vi "SET.vi"(6 "value":string, 8 "error in (no error)":errorcluster, 9 "options":T1={"ms timeout"=-1, "expire time"=timestamp(0 s since 1904-01-01), "NX"=FALSE, "XX"=FALSE, "KEEPTTL"=FALSE, "GET"=FALSE}, 10 "key":string, 11 "Redis Client in":refnum<class "Redis Client.lvclass">) -> (0 "error out":errorcluster, 1 "response":variant, 3 "Redis Client out":refnum<class "Redis Client.lvclass">)   [LabVIEW 2019, in "Redis Client for LabVIEW.lvlib" / "Redis Client.lvclass"]
uses:
  Redis Client.lvclass
  RESP3 for LabVIEW/RESP3/subVIs/RESP3 Make String Base.vi
  RESP3 for LabVIEW/RESP3/types/RESP3 data type attribute.vi
  RESP3 for LabVIEW/RESP3/high-level/RESP3 Get String.vi
  RESP3 for LabVIEW/RESP3/RESP3.lvlib
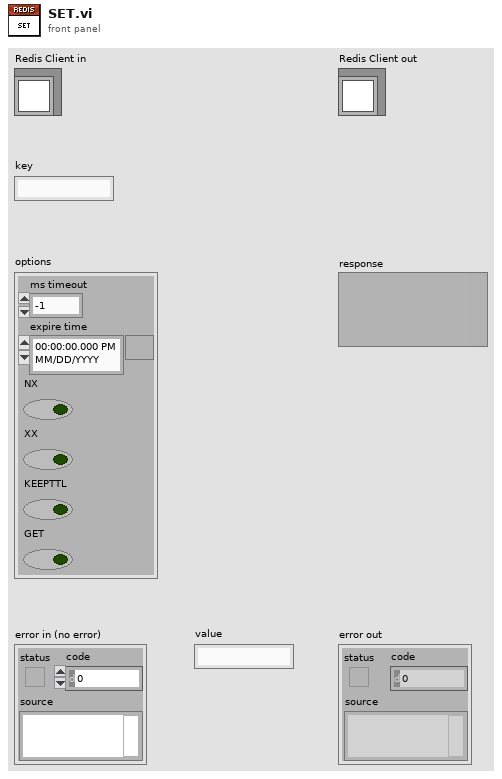
[diagram p1: front panel]
types:
  T1 = cluster{"ms timeout":i64, "expire time":timestamp, "NX":bool, "XX":bool, "KEEPTTL":bool, "GET":bool}
  T2 = typedef "RESP3.lvlib/RESP3 Type.ctl" = enum8{"<0x00>", "<0x01>", "<0x02>", "<0x03>", "<0x04>", "<0x05>", "<0x06>", "<0x07>", "<0x08>", "<0x09>", "<0x0A>", "<0x0B>", "<0x0C>", "<0x0D>", "<0x0E>", "<0x0F>", "<0x10>", "<0x11>", "<0x12>", "<0x13>", "<0x14>", "<0x15>", "<0x16>", "<0x17>", "<0x18>", "<0x19>", "<0x1A>", "<0x1B>", "<0x1C>", "<0x1D>", "<0x1E>", "<0x1F>", "\" \"", "BLOB ERROR", "\"\"\"", "BOOLEAN", "BLOB", "MAP", "\"&\"", "\"'\"", "BIG NUMBER", "\")\"", "ARRAY", "STRING", "DOUBLE", "ERROR", "END", "\"/\"", "\"0\"", "\"1\"", "\"2\"", "\"3\"", "\"4\"", "\"5\"", "\"6\"", "\"7\"", "\"8\"", "\"9\"", "INTEGER", "STREAM", "\"<\"", "VERBATIM STRING", "PUSH", "\"?\"", "\"@\"", "\"A\"", "\"B\"", "\"C\"", "\"D\"", "\"E\"", "\"F\"", "\"G\"", "\"H\"", "\"I\"", "\"J\"", "\"K\"", "\"L\"", "\"M\"", "\"N\"", "\"O\"", "\"P\"", "\"Q\"", "\"R\"", "\"S\"", "\"T\"", "\"U\"", "\"V\"", "\"W\"", "\"X\"", "\"Y\"", "\"Z\"", "\"[\"", "\"\\\"", "\"]\"", "\"^\"", "NULL", "\"`\"", "\"a\"", "\"b\"", "\"c\"", "\"d\"", "\"e\"", "\"f\"", "\"g\"", "\"h\"", "\"i\"", "\"j\"", "\"k\"", "\"l\"", "\"m\"", "\"n\"", "\"o\"", "\"p\"", "\"q\"", "\"r\"", "\"s\"", "\"t\"", "\"u\"", "\"v\"", "\"w\"", "\"x\"", "\"y\"", "\"z\"", "\"{\"", "ATTRIBUTES", "\"}\"", "SET", "<0x7F>", "<0x80>", "<0x81>", "<0x82>", "<0x83>", "<0x84>", "<0x85>", "<0x86>", "<0x87>", "<0x88>", "<0x89>", "<0x8A>", "<0x8B>", "<0x8C>", "<0x8D>", "<0x8E>", "<0x8F>", "<0x90>", "<0x91>", "<0x92>", "<0x93>", "<0x94>", "<0x95>", "<0x96>", "<0x97>", "<0x98>", "<0x99>", "<0x9A>", "<0x9B>", "<0x9C>", "<0x9D>", "<0x9E>", "<0x9F>", "<0xA0>", "<0xA1>", "<0xA2>", "<0xA3>", "<0xA4>", "<0xA5>", "<0xA6>", "<0xA7>", "<0xA8>", "<0xA9>", "<0xAA>", "<0xAB>", "<0xAC>", "<0xAD>", "<0xAE>", "<0xAF>", "<0xB0>", "<0xB1>", "<0xB2>", "<0xB3>", "<0xB4>", "<0xB5>", "<0xB6>", "<0xB7>", "<0xB8>", "<0xB9>", "<0xBA>", "<0xBB>", "<0xBC>", "<0xBD>", "<0xBE>", "<0xBF>", "<0xC0>", "<0xC1>", "<0xC2>", "<0xC3>", "<0xC4>", "<0xC5>", "<0xC6>", "<0xC7>", "<0xC8>", "<0xC9>", "<0xCA>", "<0xCB>", "<0xCC>", "<0xCD>", "<0xCE>", "<0xCF>", "<0xD0>", "<0xD1>", "<0xD2>", "<0xD3>", "<0xD4>", "<0xD5>", "<0xD6>", "<0xD7>", "<0xD8>", "<0xD9>", "<0xDA>", "<0xDB>", "<0xDC>", "<0xDD>", "<0xDE>", "<0xDF>", "<0xE0>", "<0xE1>", "<0xE2>", "<0xE3>", "<0xE4>", "<0xE5>", "<0xE6>", "<0xE7>", "<0xE8>", "<0xE9>", "<0xEA>", "<0xEB>", "<0xEC>", "<0xED>", "<0xEE>", "<0xEF>", "<0xF0>", "<0xF1>", "<0xF2>", "<0xF3>", "<0xF4>", "<0xF5>", "<0xF6>", "<0xF7>", "<0xF8>", "<0xF9>", "<0xFA>", "<0xFB>", "<0xFC>", "<0xFD>", "<0xFE>"}
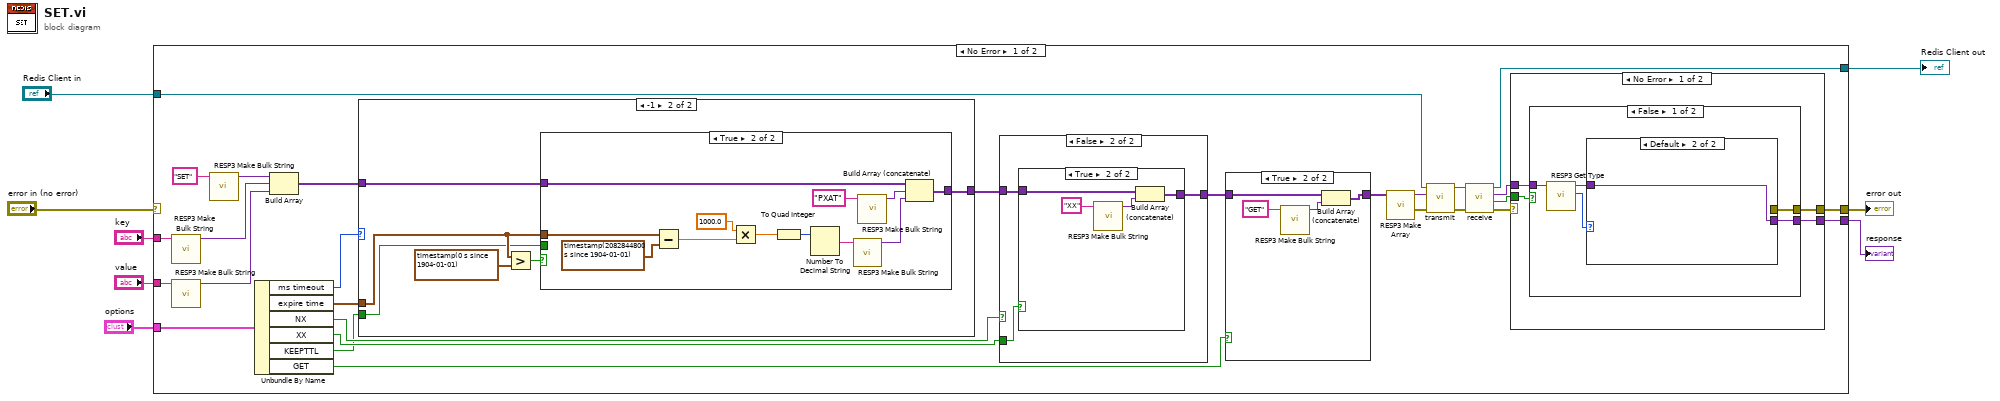
[diagram p0: block diagram]
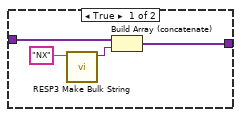
[diagram p3: hidden frame]
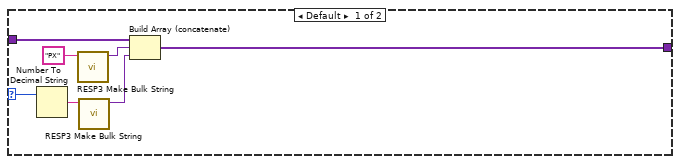
[diagram p5: hidden frame]
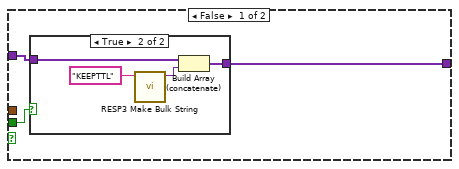
[diagram p6: hidden frame]
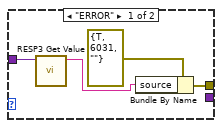
[diagram p8: hidden frame]
diagram:
  n1 = case shown="No Error" "error in (no error)" {
    selector: "error in (no error)" -> [_ w103]
    tunnel: [w29 w103] -> w7
    tunnel: "Redis Client in" -> [w36 w102]
    tunnel: [w34 w102] -> w5
    tunnel: "key" -> [w26 _]
    tunnel: [w28 _] -> w3
    tunnel: "value" -> [w21 _]
    tunnel: "options" -> [w19 _]
    frame No Error {
      n2 = call "RESP3 Make Bulk String.vi"("String"=w26) -> ("RESP3 Value out"=w24:variant)  [unwired: 9 in, 1 out]
      n3 = call "RESP3 Make Bulk String.vi"("String"=w21) -> ("RESP3 Value out"=w20:variant)  [unwired: 9 in, 1 out]
      n4 = call "RESP3 Make Bulk String.vi"("String"="SET" ("string in")) -> ("RESP3 Value out"=w25:variant)  [unwired: 9 in, 1 out]
      n5 = Unbundle By Name(w19) -> ("ms timeout"=w18:i64, "expire time"=w17:timestamp, "NX"=w15:bool, "XX"=w13:bool, "KEEPTTL"=w12:bool, "GET"=w10:bool)
      n6 = Build Array(w25, w24, w20) -> (w16:variant[])
      n7 = case shown="-1" w18 {
        selector: w18 -> [w56 _]
        tunnel: w17 -> [_ w64]
        tunnel: w16 -> [w59 w63]
        tunnel: [w54 w62] -> w14
        tunnel: w12 -> [_ w61]
        frame Default {
          n8 = Number To Decimal String(number=w56) -> (decimal integer string=w55:string)  [unwired: 1 in]
          n9 = call "RESP3 Make Bulk String.vi"("String"="PX") -> ("RESP3 Value out"=w57:variant)  [unwired: 9 in, 1 out]
          n10 = call "RESP3 Make Bulk String.vi"("String"=w55) -> ("RESP3 Value out"=w60:variant)  [unwired: 9 in, 1 out]
          n11 = Build Array (concatenate)(w59, w57, w60) -> (w54:variant[])
        }
        frame -1 {
          n12 = Greater?(x=w64, y=timestamp(0 s since 1904-01-01)) -> (0:w65:bool)
          n13 = case shown="True" w65 {
            tunnel: w64 -> [_ w85]
            tunnel: w63 -> [w68 w79]
            tunnel: [w67 w78] -> w62
            tunnel: w61 -> [w69 _]
            frame False {
              n14 = case shown="True" w69 {
                tunnel: w68 -> [w70 w72]
                tunnel: [w70 w71] -> w67
                frame False {
                }
                frame True {
                  n15 = call "RESP3 Make Bulk String.vi"("String"="KEEPTTL") -> ("RESP3 Value out"=w74:variant)  [unwired: 9 in, 1 out]
                  n16 = Build Array (concatenate)(w72, w74) -> (w71:variant[])
                }
              }
            }
            frame True {
              n17 = Subtract(x=w85, y=timestamp(2082844800 s since 1904-01-01)) -> (x-y=w84:dbl)
              n18 = Multiply(x=1000.0, y=w84) -> (x*y=w82:dbl)
              n19 = To Quad Integer(1:w82) -> (0:w75:i64)
              n20 = Number To Decimal String(number=w75) -> (decimal integer string=w81:string)  [unwired: 1 in]
              n21 = call "RESP3 Make Bulk String.vi"("String"=w81) -> ("RESP3 Value out"=w76:variant)  [unwired: 9 in, 1 out]
              n22 = call "RESP3 Make Bulk String.vi"("String"="PXAT") -> ("RESP3 Value out"=w77:variant)  [unwired: 9 in, 1 out]
              n23 = Build Array (concatenate)(w79, w77, w76) -> (w78:variant[])
            }
          }
        }
      }
      n24 = case shown="False" w15 {
        tunnel: w14 -> [w45 w48]
        tunnel: w13 -> [_ w46]
        tunnel: [w42 w47] -> w11
        frame True {
          n25 = call "RESP3 Make Bulk String.vi"("String"="NX") -> ("RESP3 Value out"=w43:variant)  [unwired: 9 in, 1 out]
          n26 = Build Array (concatenate)(w45, w43) -> (w42:variant[])
        }
        frame False {
          n27 = case shown="True" w46 {
            tunnel: w48 -> [w49 w53]
            tunnel: [w49 w50] -> w47
            frame False {
            }
            frame True {
              n28 = call "RESP3 Make Bulk String.vi"("String"="XX") -> ("RESP3 Value out"=w51:variant)  [unwired: 9 in, 1 out]
              n29 = Build Array (concatenate)(w53, w51) -> (w50:variant[])
            }
          }
        }
      }
      n30 = case shown="True" w10 {
        tunnel: w11 -> [w37 w39]
        tunnel: [w37 w38] -> w9
        frame False {
        }
        frame True {
          n31 = call "RESP3 Make Bulk String.vi"("String"="GET") -> ("RESP3 Value out"=w41:variant)  [unwired: 9 in, 1 out]
          n32 = Build Array (concatenate)(w39, w41) -> (w38:variant[])
        }
      }
      n33 = call "RESP3 Make Array.vi"("RESP3 Values in"=w9) -> ("error out"=w23:errorcluster, "RESP3 Value out"=w22:variant)  [unwired: 9 in]
      n34 = call-dynamic "transmit.vi"("error in (no error)"=w23, "RESP3 Value"=w22, "Redis Client in"=w36) -> ("error out"=w33:errorcluster, "Redis Client out"=w35:refnum<class "Redis Client.lvclass">)  [unwired: 7 in]
      n35 = call-dynamic "receive.vi"("error in (no error)"=w33, "Redis Client in"=w35) -> ("error out"=w32:errorcluster, "timed out?"=w31:bool, "RESP3 Value"=w30:variant, "Redis Client out"=w34:refnum<class "Redis Client.lvclass">)  [unwired: 6 in]
      n36 = case shown="No Error" w32 {
        selector: w32 -> [_ w101]
        tunnel: [w90 _] -> w28
        tunnel: [w89 w101] -> w29
        tunnel: w30 -> [w87 _]
        tunnel: w31 -> [w88 _]
        frame No Error {
          n37 = case shown="False" w88 {
            tunnel: [w95 _] -> w90
            tunnel: [w94 _] -> w89
            tunnel: w87 -> [w93 _]
            frame False {
              n38 = call "RESP3 Get Type.vi"("RESP3 Value in"=w93) -> ("RESP3 Type"=w91:T2, "RESP3 Value out"=w92:variant)  [unwired: 7 in, 2 out]
              n39 = case shown="Default" w91 {
                tunnel: [_ w100] -> w95
                tunnel: [w98 _] -> w94
                tunnel: w92 -> [w97 w100]
                frame "ERROR" {
                  n40 = call-poly "RESP3 Get Value.vi"("RESP3 Value in"=w97) -> ("String out"=w96:string)  [unwired: 7 in, 3 out]
                  n41 = Bundle By Name(cluster=errorcluster {"status"=TRUE, "code"=6031, "source"=""} ("error constant"), "source"=w96) -> (w98:errorcluster)
                }
                frame Default {
                }
              }
            }
            frame True {
            }
          }
        }
        frame Error {
        }
      }
    }
    frame Error {
    }
  }
  "error out" <- w7
  "Redis Client out" <- w5
  "response" <- w3
